vi "pcbPositioning.vi"() -> ()   [LabVIEW 2015]
uses:
  GlobalPath.vi
  GlobalData.vi
  GlobalVi.vi
panel:
  out "PanelName":string
  in  "?":bool
  in  "Done ?":bool
  out "Test type":string
  in  "ptfe 2":bool caption="Position the 12 PTFE pins in their dedicated holes on the reference plates"
  in  "PCB 6":bool caption="Position the PCBs on the reference plates starting from the largest one"
  in  "visual 4":bool caption="Check the PCBs for possible defects"
  in  "visual 3":bool caption="Verify that the interconnections and FEB alignment pins are mounted in position"
  in  "Table?":bool
  out "PcbFirstPart":string
  in  "stop 2":bool
  in  "Save the IDs in the database? Leave the DB open when done":bool
  in  "Fill database with all 5 PCB IDs? \nTo do this click on the PCB tab, start filling from tab 1 (1 tab per PCB), fill the \"Enter Serial/Get From DB\" box, click \"check_db\"\nThen click on the box \"Position\" ands select the PCB postition (1-5 for table and stiff1-stiff5 for the stiffback)\nThen press Add/Update \"Entry\"":bool
  in  "PCB 1":string
  in  "PCB 2":string
  in  "PCB 3":string
  in  "PCB 4":string
  in  "PCB 5":string
  # "PCB positioning on table/stiffback"
  # "(False if Stiffback)"
  # "PCB ID recording"
  # "Fill each box with the four digit PCB name\ne.g. 0030"
  # "PCB identifying through the database"
  # "Scan the ID of each of the 5 PCBs and associate them with the panel"
  # "(If the database window is closed, then click here  -->                 and load the correct panel this way: Add>Add then from the list choose \"Readout\" and then Start\n                                                                                                                                                                                                                     Choose the correct ID and click \"Start building panel\")"
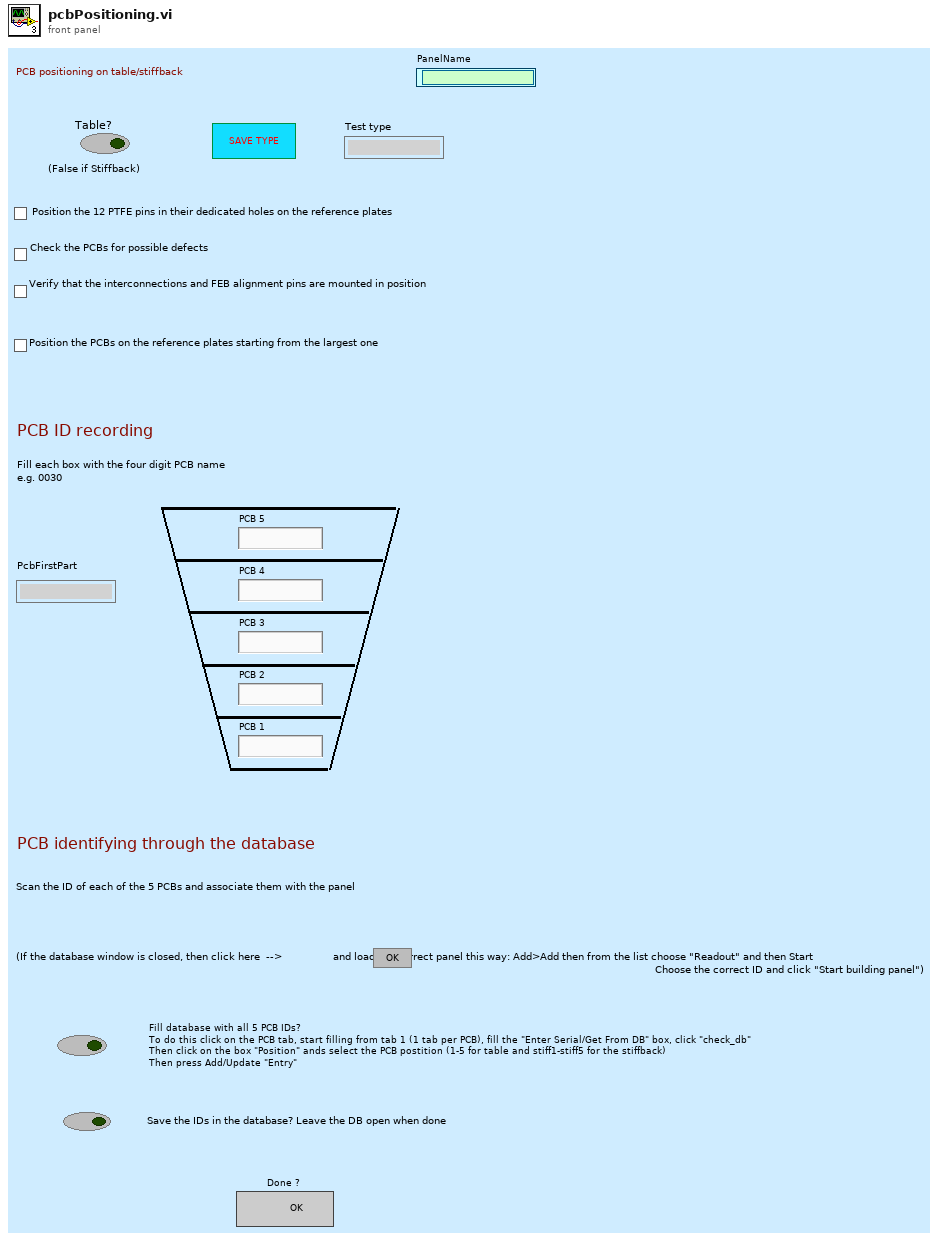
[diagram p1: front panel]
types:
  T1 = enum16{"open", "replace", "create", "open or create", "replace or create", "replace or create with confirmation"}
  T2 = enum32{"Bad", "Idle", "Run top level", "Running"}
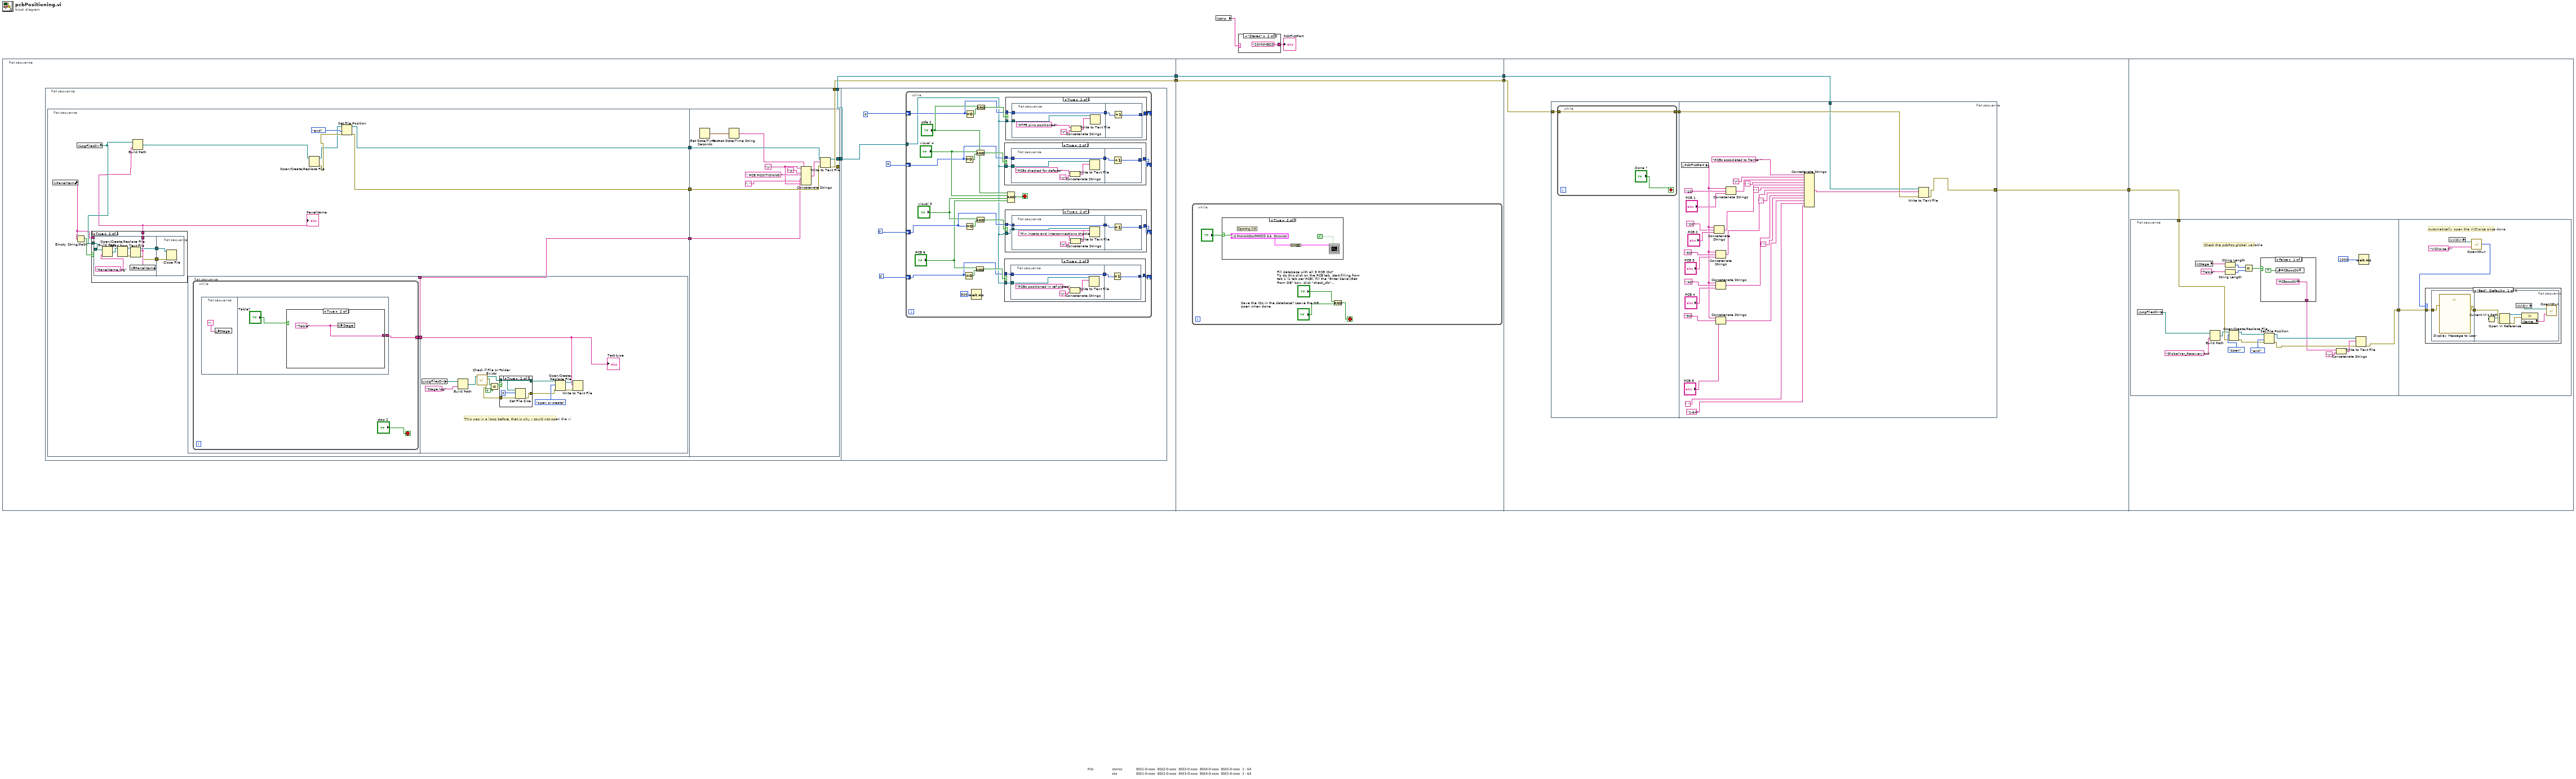
[diagram p0: block diagram]
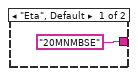
[diagram p2: hidden frame]
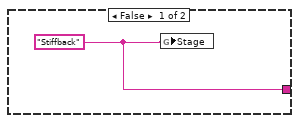
[diagram p3: hidden frame]
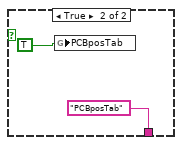
[diagram p11: hidden frame]
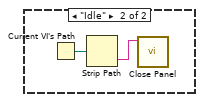
[diagram p12: hidden frame]
diagram:
  n1 = flat-sequence {
    tunnel: [w9] -> w7
    tunnel: [w8] -> w6
    tunnel: w7 -> [w160]
    tunnel: [w160] -> w2
    tunnel: w6 -> [w159]
    tunnel: [w159] -> w1
    tunnel: w2 -> [w165]
    tunnel: [w166] -> w5
    tunnel: w1 -> [w168]
    tunnel: w5 -> [w201]
    frame #0 {
      n2 = flat-sequence {
        tunnel: [w14] -> w10
        tunnel: [w14] -> w9
        tunnel: [w13] -> w8
        tunnel: w10 -> [w87]
        frame #0 {
          n3 = flat-sequence {
            tunnel: [w22] -> w15
            tunnel: [w24] -> w12
            tunnel: [w18] -> w11
            tunnel: w15 -> [w79]
            tunnel: [w78] -> w14
            tunnel: [w77] -> w13
            tunnel: w12 -> [w76]
            tunnel: w11 -> [w73]
            frame #0 {
              n4 = global read "GlobalData.vi" "PanelName"() -> (w19:string)
              n5 = Empty String/Path?(string/path=w19) -> (empty?=w21:bool)
              n6 = global read "GlobalPath.vi" "LogFilesDir"() -> (w20:path)
              n7 = case shown="True" w21 {
                tunnel: w20 -> [_ w60]
                tunnel: [w56 w59] -> w17
                tunnel: w19 -> [w56 _]
                frame False {
                }
                frame True {
                  n8 = flat-sequence {
                    tunnel: w60 -> [w68]
                    tunnel: [w63] -> w59
                    tunnel: [w62] -> w58
                    tunnel: [w61] -> w57
                    tunnel: w58 -> [w70]
                    tunnel: w57 -> [w69]
                    frame #0 {
                      n9 = Build Path(base path=w68, name or relative path="PanelName.log") -> (appended path=w67:path)
                      n10 = Open/Create/Replace File(file path (use dialog)=w67) -> (refnum out=w64:refnum<file>, error out=w65:errorcluster)  [unwired: 5 in, 1 out]
                      n11 = Read from Text File(file (use dialog)=w64, error in=w65) -> (refnum out=w61:refnum<file>, text=w63:string, error out=w62:errorcluster)  [unwired: 2 in, 1 out]
                      n12 = global write "GlobalData.vi" "PanelName"(w63) -> ()
                    }
                    frame #1 {
                      n13 = Close File(refnum=w69, error in=w70) -> ()  [unwired: 2 out]
                    }
                  }
                }
              }
              "PanelName" <- w17
              n14 = Build Path(base path=w20, name or relative path=w17) -> (appended path=w27:path)
              n15 = flat-sequence {
                tunnel: [w28] -> w18
                tunnel: [w28] -> w16
                tunnel: w16 -> [w36]
                frame #0 {
                  n16 = while {
                    tunnel: [w29] -> w28
                    stop <- "stop 2" stop-if-true
                    n17 = flat-sequence {
                      tunnel: [w32] -> w29
                      frame #0 {
                        n18 = global write "GlobalData.vi" "Stage"("") -> ()
                      }
                      frame #1 {
                        n19 = case shown="True" "Table?" {
                          tunnel: [w34 w35] -> w32
                          frame False {
                            w34 = "Stiffback"
                            n20 = global write "GlobalData.vi" "Stage"(w34) -> ()
                          }
                          frame True {
                            w35 = "Table"
                            n21 = global write "GlobalData.vi" "Stage"(w35) -> ()
                          }
                        }
                      }
                    }
                  }
                }
                frame #1 {
                  # "This was in a loop before, that is why I could not open the vi"
                  n22 = global read "GlobalPath.vi" "LogFilesDir"() -> (w40:path)
                  n23 = Build Path(base path=w40, name or relative path="Stage.log") -> (appended path=w41:path)
                  n24 = call <vilib>:"Check if File or Folder Exists.vi"("path"=w41) -> ("error out"=w46:errorcluster, "file or folder exists?"=w42:bool, "dup path"=w44:path)  [unwired: 8 in]
                  n25 = Equal?(x=w42, y=TRUE) -> (x = y?=w48:bool)
                  n26 = case shown="True" w48 {
                    tunnel: w44 -> [w51 w54]
                    tunnel: [w51 w54] -> w45
                    tunnel: [w50 w53] -> w47
                    tunnel: w46 -> [w50 w52]
                    frame False {
                    }
                    frame True {
                      n27 = Set File Size(4:w52, 6:0, 7:w54) -> (0:w53:errorcluster)  [unwired: 1 out]
                    }
                  }
                  n28 = Open/Create/Replace File(file path (use dialog)=w45, error in=w47, operation (0:open)=T1."open or create") -> (refnum out=w37:refnum<file>, error out=w38:errorcluster)  [unwired: 3 in, 1 out]
                  n29 = Write to Text File(file (use dialog)=w37, text=w36, error in=w38) -> ()  [unwired: 1 in, 3 out]
                  "Test type" <- w36
                }
              }
              n30 = Open/Create/Replace File(file path (use dialog)=w27) -> (refnum out=w23:refnum<file>, error out=w25:errorcluster)  [unwired: 5 in, 1 out]
              n31 = Set File Position(refnum=w23, from (0:start)=enum16{"start", "end", "current"}."end", error in=w25) -> (refnum out=w22:refnum<file>, error out=w24:errorcluster)  [unwired: 1 in]
            }
            frame #1 {
              w71 = "\r"
              n32 = Get Date/Time In Seconds() -> (seconds since 1Jan1904=w75:timestamp)
              n33 = Format Date/Time String(seconds (now)=w75) -> (date/time string=w74:string)  [unwired: 2 in]
              n34 = Concatenate Strings(w71, w74, "\t", " PCB POSITIONING ", w73, ": ", w71) -> (w80:string)
              n35 = Write to Text File(file (use dialog)=w79, text=w80, error in=w76) -> (refnum out=w78:refnum<file>, error out=w77:errorcluster)  [unwired: 1 in, 1 out]
            }
          }
        }
        frame #1 {
          n36 = while {
            tunnel: w87 -> [w89]
            shift-right: [w104] -> _
            shift-left: 0 -> [w105]
            shift-right: [w94] -> _
            shift-left: 0 -> [w101]
            shift-right: [w95] -> _
            shift-left: 0 -> [w97]
            shift-right: [w88] -> _
            shift-left: 0 -> [w90]
            stop <- w110 stop-if-true
            n37 = Equal To 0?(x=w90) -> (x = 0?=w93:bool)
            n38 = Equal To 0?(x=w101) -> (x = 0?=w103:bool)
            n39 = Equal To 0?(x=w97) -> (x = 0?=w99:bool)
            n40 = Equal To 0?(x=w105) -> (x = 0?=w108:bool)
            n41 = Wait (ms)(milliseconds to wait=u32 500) -> ()  [unwired: 1 out]
            n42 = And(x="PCB 6", y=w93) -> (x .and. y?=w92:bool)
            n43 = And(x="visual 4", y=w103) -> (x .and. y?=w102:bool)
            n44 = And(x="visual 3", y=w99) -> (x .and. y?=w98:bool)
            n45 = And(x="ptfe 2", y=w108) -> (x .and. y?=w106:bool)
            n46 = case shown="True" w92 {
              tunnel: w89 -> [_ w115]
              tunnel: w90 -> [w111 w113]
              tunnel: [w111 w112] -> w88
              frame False {
              }
              frame True {
                n47 = flat-sequence {
                  tunnel: w115 -> [w117]
                  tunnel: [w116] -> w114
                  tunnel: w113 -> [w116]
                  tunnel: w114 -> [w122]
                  tunnel: [w121] -> w112
                  frame #0 {
                    n48 = Concatenate Strings("PCBs positioned in ref plates", "\r") -> (w120:string)
                    n49 = Write to Text File(file (use dialog)=w117, text=w120) -> ()  [unwired: 2 in, 3 out]
                  }
                  frame #1 {
                    n50 = Increment(x=w122) -> (x+1=w121:i32)
                  }
                }
              }
            }
            n51 = case shown="True" w102 {
              tunnel: w89 -> [_ w139]
              tunnel: w101 -> [w135 w137]
              tunnel: [w135 w136] -> w94
              frame False {
              }
              frame True {
                n52 = flat-sequence {
                  tunnel: w139 -> [w141]
                  tunnel: [w140] -> w138
                  tunnel: w137 -> [w140]
                  tunnel: w138 -> [w146]
                  tunnel: [w145] -> w136
                  frame #0 {
                    n53 = Concatenate Strings("PCBs checked for defects", "\r") -> (w144:string)
                    n54 = Write to Text File(file (use dialog)=w141, text=w144) -> ()  [unwired: 2 in, 3 out]
                  }
                  frame #1 {
                    n55 = Increment(x=w146) -> (x+1=w145:i32)
                  }
                }
              }
            }
            n56 = case shown="True" w98 {
              tunnel: w89 -> [_ w127]
              tunnel: w97 -> [w123 w125]
              tunnel: [w123 w124] -> w95
              frame False {
              }
              frame True {
                n57 = flat-sequence {
                  tunnel: w127 -> [w129]
                  tunnel: [w128] -> w126
                  tunnel: w125 -> [w128]
                  tunnel: w126 -> [w134]
                  tunnel: [w133] -> w124
                  frame #0 {
                    n58 = Concatenate Strings("Pin inserts and interconnections checked", "\r") -> (w132:string)
                    n59 = Write to Text File(file (use dialog)=w129, text=w132) -> ()  [unwired: 2 in, 3 out]
                  }
                  frame #1 {
                    n60 = Increment(x=w134) -> (x+1=w133:i32)
                  }
                }
              }
            }
            n61 = case shown="True" w106 {
              tunnel: w89 -> [_ w151]
              tunnel: w105 -> [w147 w149]
              tunnel: [w147 w148] -> w104
              frame False {
              }
              frame True {
                n62 = flat-sequence {
                  tunnel: w151 -> [w153]
                  tunnel: [w152] -> w150
                  tunnel: w149 -> [w152]
                  tunnel: w150 -> [w158]
                  tunnel: [w157] -> w148
                  frame #0 {
                    n63 = Concatenate Strings("PTFE pins positioned", "\r") -> (w156:string)
                    n64 = Write to Text File(file (use dialog)=w153, text=w156) -> ()  [unwired: 2 in, 3 out]
                  }
                  frame #1 {
                    n65 = Increment(x=w158) -> (x+1=w157:i32)
                  }
                }
              }
            }
            n66 = Compound Arithmetic op=AND("ptfe 2", "visual 4", "visual 3", "PCB 6") -> (w110:bool)
          }
        }
      }
    }
    frame #1 {
      n67 = while {
        stop <- w162 stop-if-true
        n68 = case shown="True" "?" {
          frame False {
          }
          frame True {
          }
        }
        n69 = And(x="Fill database with all 5 PCB IDs? \nTo do this click on the PCB tab, start filling from tab 1 (1 tab per PCB), fill the \"Enter Serial/Get From DB\" box, click \"check_db\"\nThen click on the box \"Position\" ands select the PCB postition (1-5 for table and stiff1-stiff5 for the stiffback)\nThen press Add/Update \"Entry\"", y="Save the IDs in the database? Leave the DB open when done") -> (x .and. y?=w162:bool)
      }
    }
    frame #2 {
      n70 = flat-sequence {
        tunnel: w168 -> [w170]
        tunnel: [w169] -> w167
        tunnel: w167 -> [w175]
        tunnel: [w173] -> w166
        tunnel: w165 -> [w174]
        frame #0 {
          n71 = while {
            tunnel: w170 -> [w171]
            tunnel: [w171] -> w169
            stop <- "Done ?" stop-if-true
          }
        }
        frame #1 {
          n72 = local read "PcbFirstPart"() -> (w176:string)
          n73 = Concatenate Strings(w176, "20", "PCB 2") -> (w186:string)
          n74 = Concatenate Strings(w176, "30", "PCB 3") -> (w184:string)
          n75 = Concatenate Strings(w176, "40", "PCB 4") -> (w182:string)
          n76 = Concatenate Strings(w176, "50", "PCB 5") -> (w180:string)
          n77 = Concatenate Strings(w176, "10", "PCB 1") -> (w188:string)
          n78 = Concatenate Strings("PCBs associated to frame: ", "\r", w188, " ", w186, " ", w184, " ", w182, " ", w180, " ", "1-64") -> (w177:string)
          n79 = Write to Text File(file (use dialog)=w174, text=w177, error in=w175) -> (error out=w173:errorcluster)  [unwired: 1 in, 2 out]
        }
      }
    }
    frame #3 {
      n80 = flat-sequence {
        tunnel: [w203] -> w202
        tunnel: w201 -> [w207]
        tunnel: w202 -> [w227]
        frame #0 {
          # "Check the pcbPos global variable"
          n81 = global read "GlobalPath.vi" "LogFilesDir"() -> (w205:path)
          n82 = global read "GlobalData.vi" "Stage"() -> (w218:string)
          n83 = Build Path(base path=w205, name or relative path="GlobalVar_Recovery.txt") -> (appended path=w216:path)
          n84 = String Length(string=w218) -> (length=w220:i32)
          n85 = String Length(string="Table") -> (length=w221:i32)
          n86 = Open/Create/Replace File(file path (use dialog)=w216, error in=w207, operation (0:open)=T1."open") -> (refnum out=w212:refnum<file>, error out=w213:errorcluster)  [unwired: 3 in, 1 out]
          n87 = Equal?(x=w220, y=w221) -> (x = y?=w222:bool)
          n88 = case shown="False" w222 {
            tunnel: ["PCBposStiff" "PCBposTab"] -> w206
            frame False {
              n89 = global write "GlobalVi.vi" "PCBposStiff"(TRUE) -> ()
            }
            frame True {
              n90 = global write "GlobalVi.vi" "PCBposTab"(TRUE) -> ()
            }
          }
          n91 = Set File Position(refnum=w212, from (0:start)=enum16{"start", "end", "current"}."end", error in=w213) -> (refnum out=w209:refnum<file>, error out=w208:errorcluster)  [unwired: 1 in]
          n92 = Concatenate Strings(w206, "\r") -> (w211:string)
          n93 = Write to Text File(file (use dialog)=w209, text=w211, error in=w208) -> (error out=w203:errorcluster)  [unwired: 1 in, 2 out]
          n94 = Wait (ms)(milliseconds to wait=1000) -> ()  [unwired: 1 out]
        }
        frame #1 {
          # "Automatically open the ViChoice once done"
          n95 = global read "GlobalPath.vi" "ViDir"() -> (w230:path)
          n96 = call "OpenNRun.vi"("VI name"="ViChoice.vi", "ViDirPath"=w230) -> ("Execution:State"=w229:T2)
          n97 = case shown="\"Bad\", Default" w229 {
            tunnel: w227 -> [w232 _]
            frame "Bad", Default {
              n98 = flat-sequence {
                tunnel: w232 -> [w234]
                tunnel: [w233] -> w231
                tunnel: w231 -> [w236]
                frame #0 {
                  n99 = call "Display Message to User"("error in (no error)"=w234) -> ("error out"=w233:errorcluster)  [unwired: 9 in, 1 out]
                }
                frame #1 {
                  n100 = Current VI's Path() -> (path=w235:path)
                  n101 = Open VI Reference(vi path=w235, error in (no error)=w236) -> (vi reference=w240:refnum<vi>, error out=w239:errorcluster)  [unwired: 4 in]
                  n102 = global read "GlobalPath.vi" "ViDir"() -> (w238:path)
                  n103 = property class="VI"(reference=w240, error in=w239) -> ("Name"=w237:string)  [unwired: 2 out]
                  n104 = call "OpenNRun.vi"("VI name"=w237, "ViDirPath"=w238) -> ()  [unwired: 1 out]
                }
              }
            }
            frame "Idle" {
              n105 = Current VI's Path() -> (path=w241:path)
              n106 = Strip Path(path=w241) -> (name=w242:string)  [unwired: 1 out]
              n107 = call <vilib>:"Close Panel.vi"("VI name"=w242) -> ()  [unwired: 10 in, 1 out]
            }
          }
        }
      }
    }
  }
  n108 = global read "GlobalData.vi" "strip"() -> (w4:string)
  n109 = case shown="\"Stereo\"" w4 {
    tunnel: ["20MNMBSE" "20MNMBSS"] -> w3
    frame "Eta", Default {
    }
    frame "Stereo" {
    }
  }
  "PcbFirstPart" <- w3
